vi "Annealing.vi"() -> ()   [LabVIEW 2020]
uses:
  <vilib>/Analysis/1siggen.llb/Ramp Pattern by Delta.vi
  <vilib>/Analysis/NI_AALBase.lvlib
  AnnealingDriver/Agilent E363X Series/Agilent E363X Series.lvlib
panel:
  in  "Hold Time (h)":dbl
  in  "Voltage Limit (V)":dbl=1.0 format="%.3g"
  in  "VISA resource name":refnum<visa-resource-name>
  out "?":cluster{"Y":dbl[], "Y":dbl[]}[](graph)
  out "Elapsed Time (min)":dbl
  out "Total Time (min)":dbl
  out "Total Steps":dbl
  out "Elapsed Steps":dbl
  out "Current Now (A)":dbl
  in  "Step Time (s)":dbl
  in  "Step Size (A)":dbl
  in  "End (A)":dbl
  in  "Start (A)":dbl
  # "Annealing Current Control"
  # "1. Ramps up from Start to End with Step Size and Step Time. \n2. Holds at End for Hold Time. \n3. Ramps down from End to Start with Step Size and Step Time.\n\n\nSelect \"Run\" (not \"Run Continously\") to turn voltage output \noff once ramp down is complete. \n\nEnter Device details and Parameters before pressing \"Run\".\nHardware: Agilent Hewlett-Packard E3631A"
  # "Parameters"
  # "Progress"
  # "Device"
  # "Seconds!"
  # "Hours!"
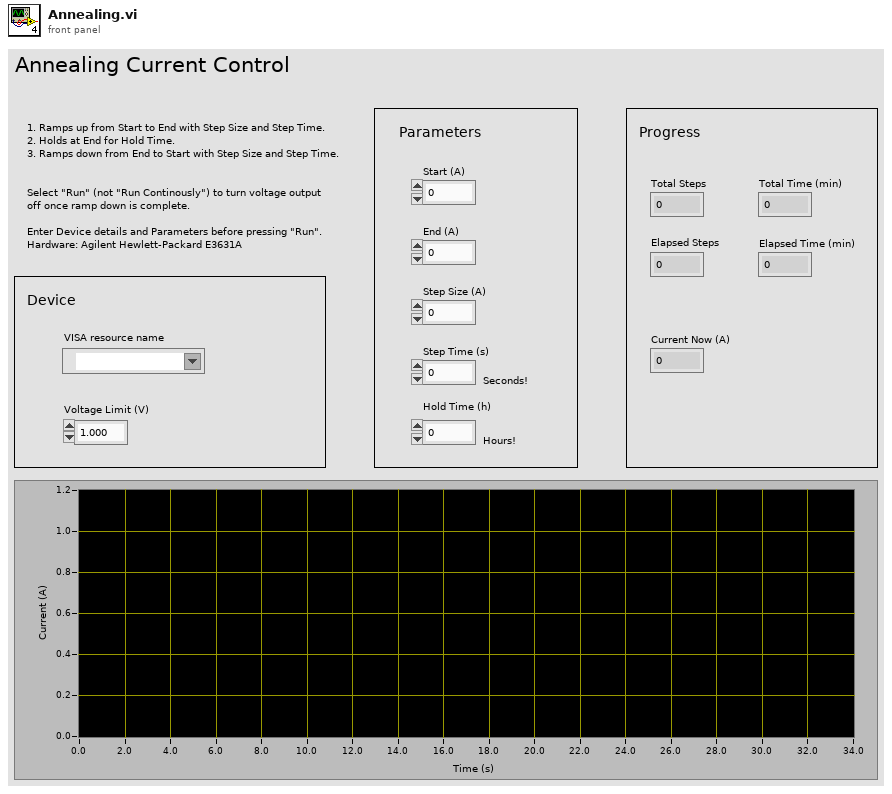
[diagram p1: front panel]
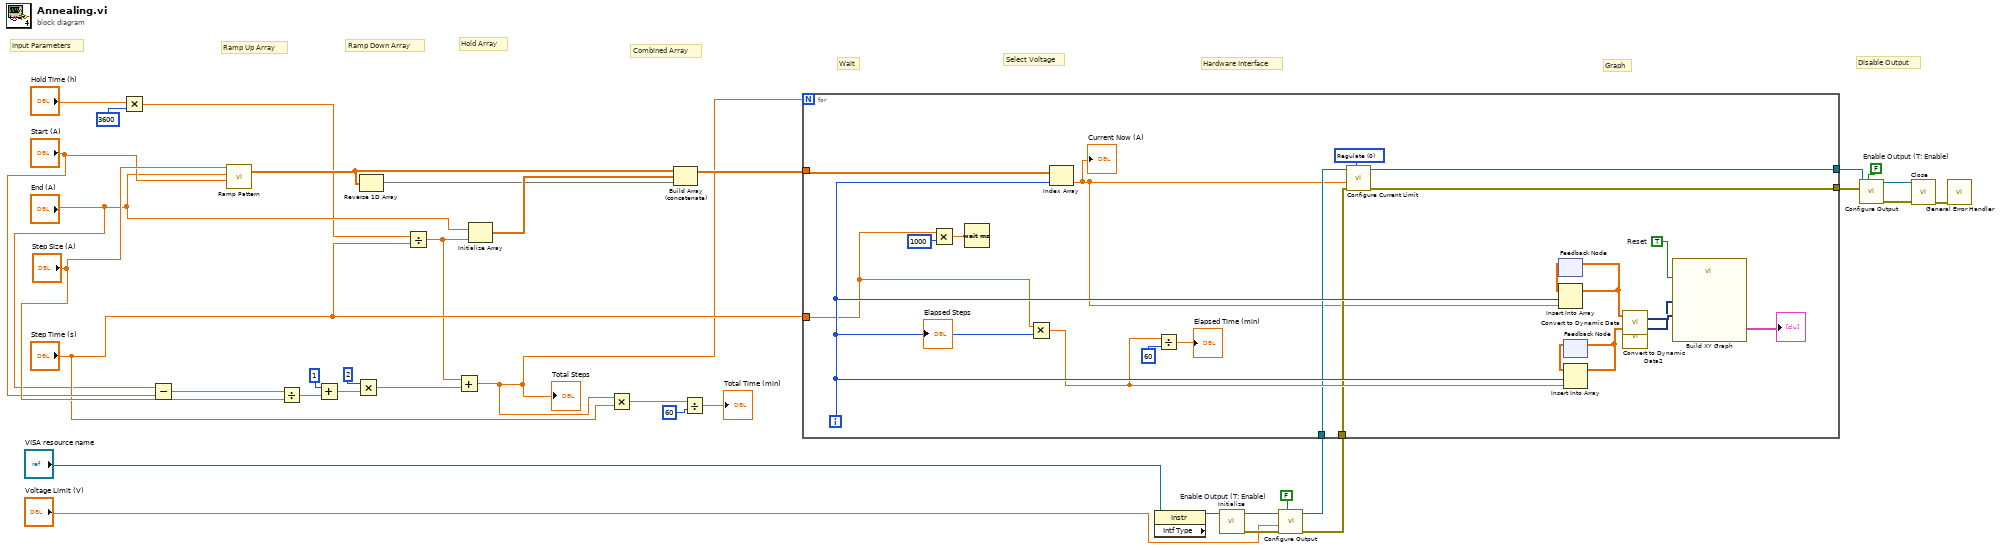
[diagram p0: block diagram]
diagram:
  w8 = FALSE  # Enable Output (T: Enable)
  w32 = FALSE  # Enable Output (T: Enable)
  # "Combined Array"
  # "Hold Array"
  # "Ramp Down Array"
  # "Graph"
  # "Hardware Interface"
  # "Disable Output"
  # "Select Voltage"
  # "Wait"
  # "Ramp Up Array"
  # "Input Parameters"
  n1 = Multiply(x="Hold Time (h)", y=3600) -> (x*y=w13:dbl)
  n2 = Subtract(x="End (A)", y="Start (A)") -> (x-y=w36:dbl)
  n3 = call-poly <vilib>:"Ramp Pattern.vi"("start"="Start (A)", "end"="End (A)", "delta"="Step Size (A)") -> ("Ramp Pattern"=w24:dbl[])  [unwired: 6 in, 2 out]
  n4 = Divide(x=w36, y="Step Size (A)") -> (x/y=w19:dbl)
  n5 = Add(x=1, y=w19) -> (x+y=w18:dbl)
  n6 = Multiply(x=2, y=w18) -> (x*y=w16:dbl)
  n7 = Reverse 1D Array(array=w24) -> (reversed array=w20:dbl[])
  n8 = Divide(x=w13, y="Step Time (s)") -> (x/y=w15:dbl)
  n9 = Add(x=w15, y=w16) -> (x+y=w5:dbl)
  "Total Steps" <- w5
  n10 = Initialize Array("End (A)", w15) -> (w21:dbl[])
  n11 = Multiply(x=w5, y="Step Time (s)") -> (x*y=w11:dbl)
  n12 = Build Array (concatenate)(w24, w21, w20) -> (w26:dbl[])
  n13 = Divide(x=w11, y=60) -> (x/y=→"Total Time (min)":dbl)
  n14 = property class="Instr" props=["Intf Type"](reference="VISA resource name") -> (reference out=w29:refnum<visa-resource-name>)  [unwired: 1 in, 2 out]
  n15 = call "Initialize.vi"("VISA resource name"=w29) -> ("error out"=w6:errorcluster, "VISA resource name out"=w7:refnum<visa-resource-name>)  [unwired: 9 in]
  n16 = call "Configure Output.vi"("Enable Output (T: Enable)"=w8, "error in (no error)"=w6, "Voltage Level (0.0 V)"="Voltage Limit (V)", "VISA resource name"=w7) -> ("error out"=w1:errorcluster, "VISA resource name out"=w2:refnum<visa-resource-name>)  [unwired: 6 in]
  n17 = for {
    N: w5 -> [_]
    tunnel: "Step Time (s)" -> [w49]
    tunnel: w26 -> [w58]
    tunnel: [w40] -> w31
    tunnel: [w41] -> w30
    tunnel: w1 -> [w45]
    tunnel: w2 -> [w44]
    i -> [w50]
    w39 = TRUE  # Reset
    w43 = u16 0 items=["Regulate", "Trip"] ("Behavior (0: Regulate)")
    n18 = Multiply(x=w49, y=1000) -> (x*y=w52:dbl)
    n19 = Wait (ms)(milliseconds to wait=w52) -> ()  [unwired: 1 out]
    n20 = Multiply(x=w49, y=w50) -> (x*y=w47:dbl)
    n21 = Index Array(array=w58, index=w50) -> (element=w42:dbl)
    "Current Now (A)" <- w42
    n22 = Divide(x=w47, y=60) -> (x/y=→"Elapsed Time (min)":dbl)
    n23 = call "Configure Current Limit.vi"("Behavior (0: Regulate)"=w43, "error in (no error)"=w45, "Current Limit (0.0 A)"=w42, "VISA resource name"=w44) -> ("error out"=w40:errorcluster, "VISA resource name out"=w41:refnum<visa-resource-name>)  [unwired: 6 in]
    n24 = feedback #1() -> (w56:dbl[])  [unwired: 1 in]
    n25 = Insert Into Array(array=w56, index=w50, new element=w42) -> (w38:dbl[])
    n26 = feedback-in #1(w38) -> ()
    n27 = feedback #2() -> (w55:dbl[])  [unwired: 1 in]
    n28 = Insert Into Array(array=w55, index=w50, new element=w47) -> (w37:dbl[])
    n29 = feedback-in #2(w37) -> ()
    n30 = call "Convert to Dynamic Data"("Array"=w38) -> ("Dynamic Data Type"=w54:dynamicdata)  [unwired: 3 in]
    n31 = call "Convert to Dynamic Data2"("Array"=w37) -> ("Dynamic Data Type"=w53:dynamicdata)  [unwired: 3 in]
    n32 = call "Build XY Graph"("Reset"=w39, "Y Input"=w54, "X Input"=w53) -> ("XY Graph"=→"?":cluster{"X":dbl[], "Y":dbl[]}[])  [unwired: 7 in, 1 out]
    "Elapsed Steps" <- w50
  }
  n33 = call "Configure Output.vi"("Enable Output (T: Enable)"=w32, "error in (no error)"=w31, "VISA resource name"=w30) -> ("error out"=w33:errorcluster, "VISA resource name out"=w34:refnum<visa-resource-name>)  [unwired: 7 in]
  n34 = call "Close.vi"("error in (no error)"=w33, "VISA resource name"=w34) -> ("error out"=w35:errorcluster)  [unwired: 9 in]
  n35 = call <vilib>:"General Error Handler.vi"("error in (no error)"=w35) -> ()  [unwired: 10 in, 5 out]
